vi "Tx End.vi"(8 "error in":errorcluster, 11 "performance in":refnum<class "Performance.lvclass">) -> (0 "error out":errorcluster, 3 "performance out":refnum<class "Performance.lvclass">)   [LabVIEW 2019, in "DSF Core.lvlib" / "Performance.lvclass"]
uses:
  Performance.lvclass
  Performance.lvclass/Performance.ctl
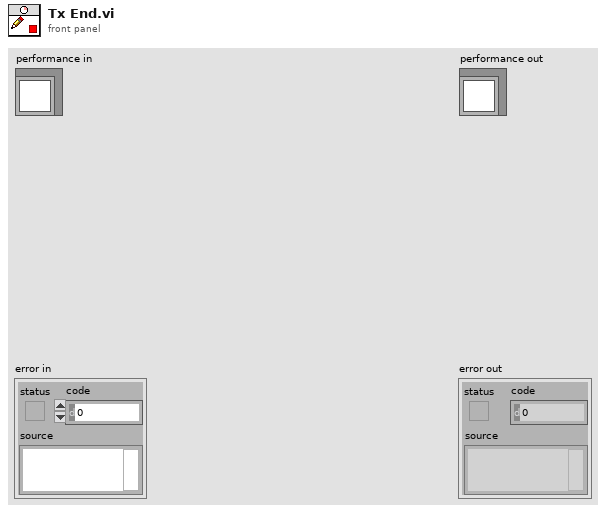
[diagram p1: front panel]
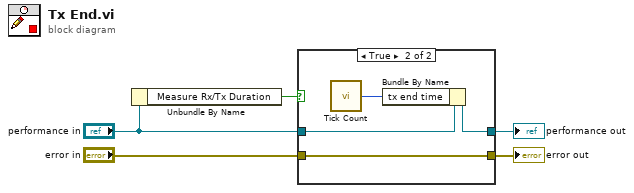
[diagram p0: block diagram]
diagram:
  n1 = Unbundle By Name("performance in") -> ("Measure Rx/Tx Duration"=w1:bool)
  n2 = case shown="True" w1 {
    tunnel: [w6 w11] -> w5
    tunnel: "error in" -> [w6 w11]
    tunnel: [w7 w8] -> w3
    tunnel: "performance in" -> [w7 w9]
    frame False {
    }
    frame True {
      n3 = call "Tick Count"() -> ("Tick Count(uSec)"=w10:u32)
      n4 = Bundle By Name(cluster=w9, "tx end time"=w10) -> (w8:refnum<class "Performance.lvclass">)
    }
  }
  "error out" <- w5
  "performance out" <- w3
